vi "SetFurniture.vi"(8 "error in (no error)":errorcluster, 10 "Furniture":refnum<class "Furniture.lvclass">[](array[class]), 11 "Room in":refnum<class "Room.lvclass">) -> (0 "error out":errorcluster, 3 "Room out":refnum<class "Room.lvclass">)   [LabVIEW 2019, in "Room.lvclass"]
uses:
  Room.lvclass
  Furniture.lvclass
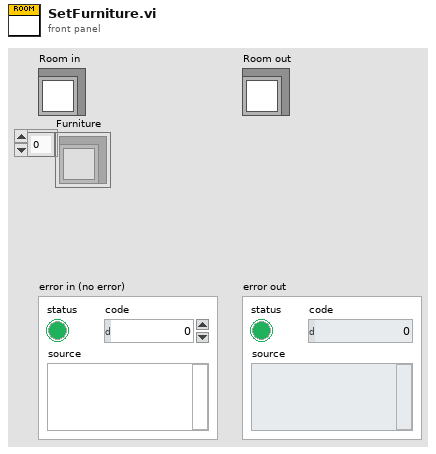
[diagram p1: front panel]
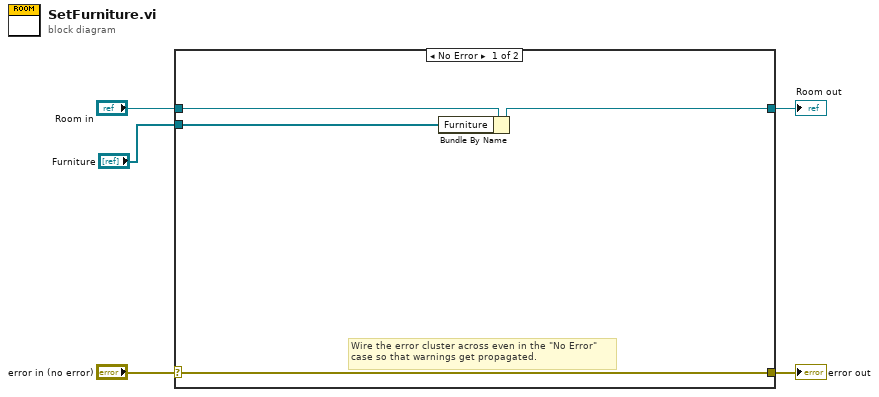
[diagram p0: block diagram]
diagram:
  n1 = case shown="No Error" "error in (no error)" {
    selector: "error in (no error)" -> [w8 w11]
    tunnel: [w8 w11] -> w2
    tunnel: [w7 w10] -> w4
    tunnel: "Room in" -> [w9 w10]
    tunnel: "Furniture" -> [w6 _]
    frame No Error {
      # "Wire the error cluster across even in the \"No Error\"\ncase so that warnings get propagated."
      n2 = Bundle By Name(cluster=w9, "Furniture"=w6) -> (w7:refnum<class "Room.lvclass">)
    }
    frame Error {
    }
  }
  "Room out" <- w4
  "error out" <- w2
